vi "ELVIS III v1.0 Unreserve Channel.vi"(5 "Allow multiple opens?":bool, 7 "Owner":string, 8 "error in (no error)":errorcluster, 9 "Mutex IDS":u32[](array[numeric]), 10 "Connector":T1=enum."ConnectorB", 11 "Channel Name":string) -> (0 "error out":errorcluster)   [LabVIEW 2021]
uses:
  <vilib>/myRIO/Common/Instrument Driver Framework/ELVIS III v1.0/Resource Manager/typedefs/ELVIS III v1.0 Connector List.ctl
  <vilib>/myRIO/Common/Instrument Driver Framework/Utilities/typedefs/Resource Manager Action Enum.ctl
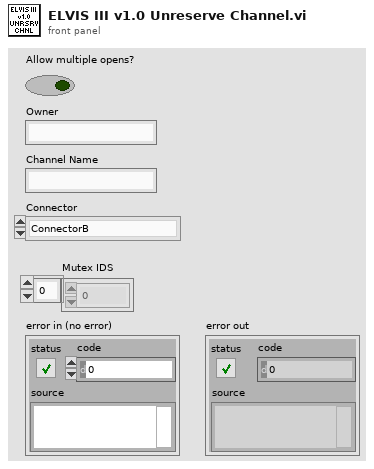
[diagram p1: front panel]
types:
  T1 = typedef "ELVIS III v1.0 Connector List.ctl" = enum32{"None", "ConnectorA", "ConnectorB"}
  T2 = typedef "Resource Manager Action Enum.ctl" = enum16{"Lock", "Unlock"}
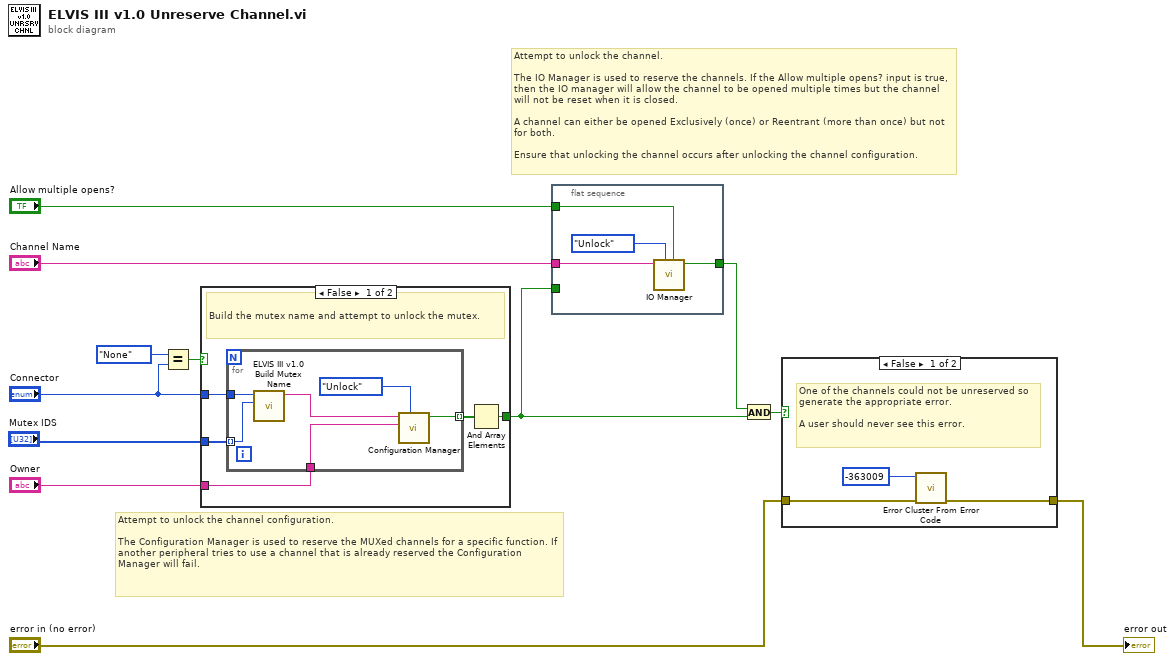
[diagram p0: block diagram]
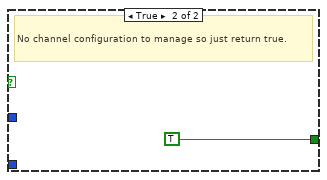
[diagram p3: hidden frame]
diagram:
  # "Attempt to unlock the channel configuration.\n\nThe Configuration Manager is used to reserve the MUXed channels for a specific function. If another peripheral tries to use a channel that is already reserved the Configuration Manager will fail."
  # "Attempt to unlock the channel.\n\nThe IO Manager is used to reserve the channels. If the Allow multiple opens? input is true, then the IO manager will allow the channel to be opened multiple times but the channel will not be reset when it is closed.\n\nA channel can either be opened Exclusively (once) or Reentrant (more than once) but not for both.\n\nEnsure that unlocking the channel occurs after unlocking the channel configuration."
  n1 = Equal?(x=ELVIS_III_v1.0_Connector_List."None" ("Connector"), y="Connector") -> (x = y?=w8:bool)
  n2 = case shown="False" w8 {
    tunnel: [w13 TRUE ("Reentrant?")] -> w6
    tunnel: "Owner" -> [w17 _]
    tunnel: "Connector" -> [w16 _]
    tunnel: "Mutex IDS" -> [w15 _]
    frame False {
      # "Build the mutex name and attempt to unlock the mutex."
      n3 = for {
        tunnel: w17 -> [w23]
        tunnel: [w21] -> w14 mode=indexing
        tunnel: w16 -> [w20]
        tunnel: w15 -> [w19] mode=indexing
        n4 = call <vilib>:"ELVIS III v1.0 Build Mutex Name.vi"("Mutex ID"=w19, "Connector"=w20) -> ("Mutex Name"=w18:string)  [unwired: 9 in]
        n5 = call <vilib>:"Configuration Manager.vi"("Actions"=Resource_Manager_Action_Enum."Unlock", "Owner"=w23, "Mutex Name"=w18) -> ("Success?"=w21:bool)  [unwired: 8 in]
      }
      n6 = And Array Elements(Boolean array=w14) -> (logical AND=w13:bool)
    }
    frame True {
      # "No channel configuration to manage so just return true."
    }
  }
  n7 = flat-sequence {
    tunnel: "Allow multiple opens?" -> [w28]
    tunnel: "Channel Name" -> [w27]
    tunnel: [w26] -> w7
    tunnel: w6 -> [_]
    frame #0 {
      n8 = call <vilib>:"IO Manager.vi"("Reentrant?"=w28, "Actions"=Resource_Manager_Action_Enum."Unlock", "Mutex Name"=w27) -> ("Success?"=w26:bool)  [unwired: 8 in]
    }
  }
  n9 = And(x=w7, y=w6) -> (x .and. y?=w5:bool)
  n10 = case shown="False" w5 {
    tunnel: "error in (no error)" -> [w31 w32]
    tunnel: [w30 w32] -> w3
    frame False {
      # "One of the channels could not be unreserved so generate the appropriate error.\n\nA user should never see this error."
      n11 = call <vilib>:"Error Cluster From Error Code.vi"("error in (no error)"=w31, "error code (0)"=-363009) -> ("error out"=w30:errorcluster)  [unwired: 7 in]
    }
    frame True {
    }
  }
  "error out" <- w3
